vi "ReadHeader.vi"(8 "name":string, 9 "[A] name":string[](array[string]), 10 "End":u32[](array[numeric]), 11 "Start":u32[](array[numeric])) -> (1 "End":u32, 2 "Start":u32)   [LabVIEW 2017, in "HEKAdat.lvclass"]
uses:
  HEKAdat.lvclass
panel:
  out "index of element":i32
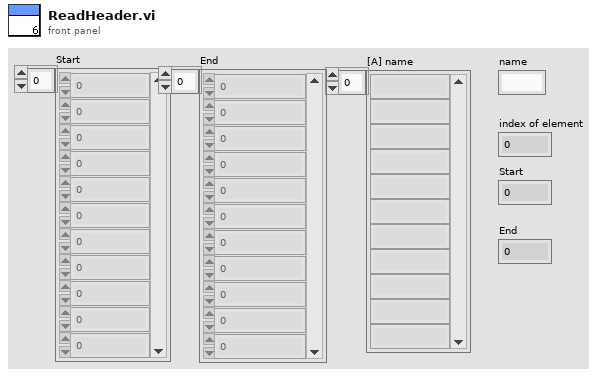
[diagram p1: front panel]
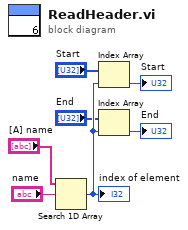
[diagram p0: block diagram]
diagram:
  n1 = Search 1D Array(1D array="[A] name", element="name") -> (index of element=w6:i32)  [unwired: 1 in]
  "index of element" <- w6
  n2 = Index Array(array="Start", index=w6) -> (element=→"Start":u32)
  n3 = Index Array(array="End", index=w6) -> (element=→"End":u32)
